vi "AI 20kHz data FGV.vi"(8 "error in":errorcluster, 10 "Enum":enum16{"Read", "Write"}(ring), 11 "Propulsion Data":dbl[](array[numeric])) -> (0 "error out":errorcluster, 3 "Propulsion Data":dbl[](array[numeric]))   [LabVIEW 2022 SP3]
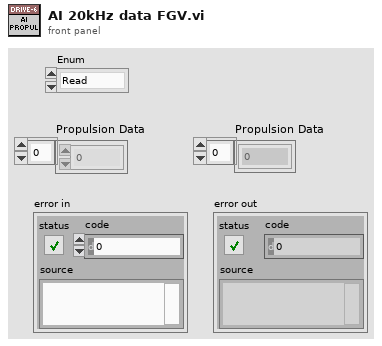
[diagram p1: front panel]
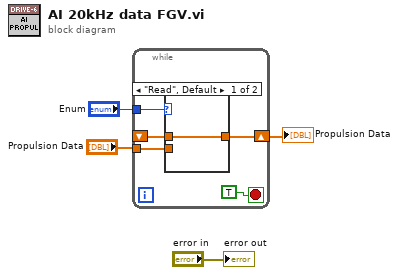
[diagram p0: block diagram]
diagram:
  n1 = while {
    tunnel: "Enum" -> [w9]
    tunnel: "Propulsion Data" -> [w7]
    shift-right: [w6] -> w1
    shift-left: _ -> [w5]
    stop <- TRUE stop-if-true
    n2 = case shown="\"Read\", Default" w9 {
      tunnel: w7 -> [_ w11]
      tunnel: [w10 w11] -> w6
      tunnel: w5 -> [w10 _]
      frame "Read", Default {
      }
      frame "Write" {
      }
    }
  }
  "Propulsion Data" <- w1
  "error out" <- "error in"
